vi "SetRampRates_ReadField.vi"(0 "Max Ramp Rate - Z Axis (A/s)":dbl, 1 "Max Ramp Rate - Y Axis (A/s)":dbl, 2 "User defined Ramp Rate (T/min) 2":bool, 3 "User defined Ramp Rate (T/min)":dbl, 5 "Within Limits?":bool, 7 "Y-Axis Field (kG)":dbl, 9 "Z-Axis Field (kG) in":dbl, 11 "error in (no error)":T1, 12 "Y-Axis Communications Config":T2, 13 "Z-Axis Communications Config":T2) -> (4 "All Instruments Responded?":bool, 6 "Current Magnetic\nField\n(430 TCP reading)":T3 {"phi (deg)" format="%#_3g"}, 8 "Ramp Rate along Vector (T/min)":dbl, 10 "Y-Axis Ramp Rate (T/min)":dbl format="%.3f", 14 "Z-Axis Ramp Rate (T/min)":dbl format="%.3f", 15 "error out":T1)   [LabVIEW 2013]
uses:
  VTI LabView IS - Kopie2/devices/magnet/AMI reading polar field.ctl
  VTI LabView IS - Kopie2/app/app global state actions.ctl
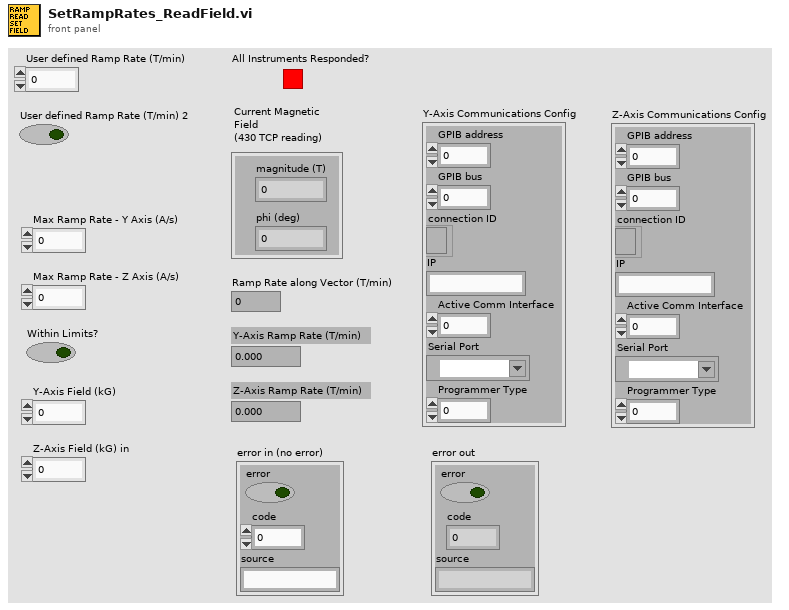
[diagram p1: front panel]
types:
  T1 = cluster{"error":bool, "code":i32, "source":string}
  T2 = cluster{"GPIB address":i16, "GPIB bus":i16, "connection ID":refnum<k5>, "IP":string, "Active Comm Interface":u16, "Serial Port":refnum<visa-resource-name>, "Programmer Type":u16}
  T3 = typedef "AMI reading polar field.ctl" = cluster{"magnitude (T)":dbl, "phi (deg)":dbl}
  T4 = typedef "app global state actions.ctl" = enum16{"set field reached", "get cluster", "set cluster", "set current sweep", "set field value", "set 430 TCP reading", "set ramping", "set sweeping", "append log", "clear log", "set finished"}
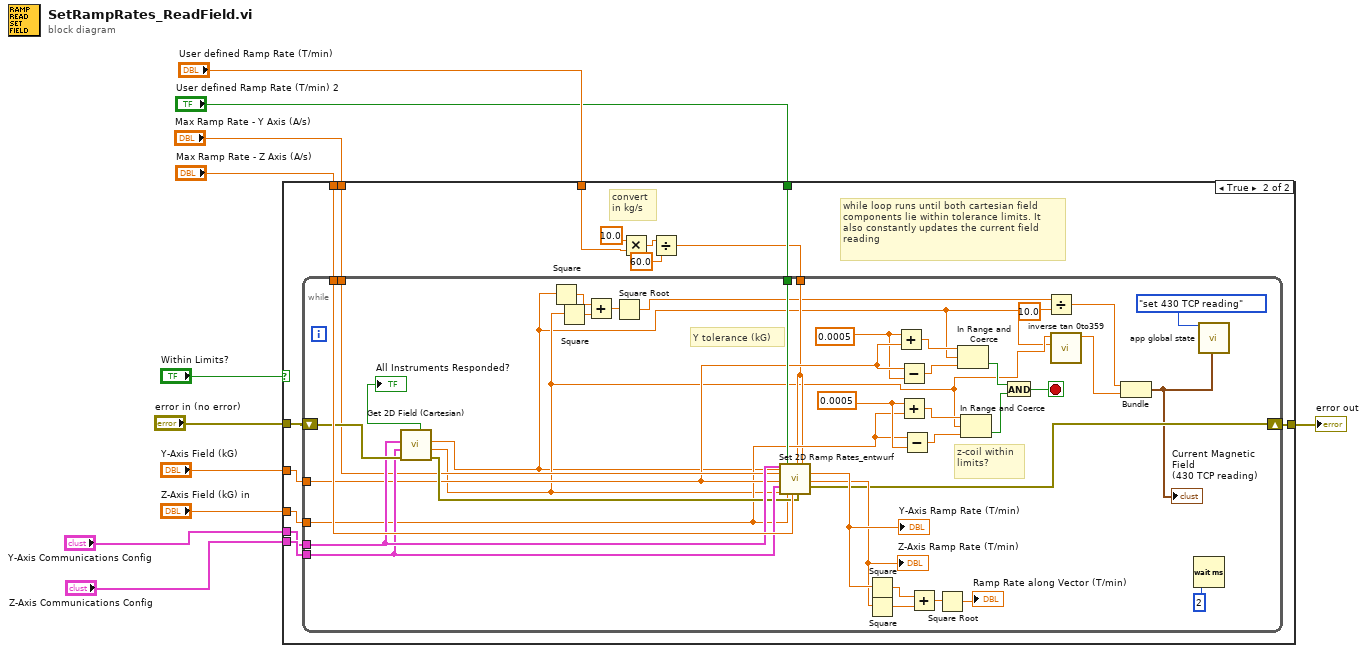
[diagram p0: block diagram]
diagram:
  n1 = case shown="True" "Within Limits?" {
    tunnel: "Z-Axis Field (kG) in" -> [_ w26]
    tunnel: "Y-Axis Field (kG)" -> [_ w25]
    tunnel: [w12 w24] -> w4
    tunnel: "User defined Ramp Rate (T/min) 2" -> [_ w23]
    tunnel: "Max Ramp Rate - Y Axis (A/s)" -> [_ w22]
    tunnel: "Max Ramp Rate - Z Axis (A/s)" -> [_ w21]
    tunnel: "error in (no error)" -> [w12 w20]
    tunnel: "Z-Axis Communications Config" -> [_ w19]
    tunnel: "Y-Axis Communications Config" -> [_ w18]
    tunnel: "User defined Ramp Rate (T/min)" -> [_ w14]
    frame False {
    }
    frame True {
      # "convert \nin kg/s"
      # "while loop runs until both cartesian field components lie within tolerance limits. It also constantly updates the current field reading"
      n2 = Multiply(x=10.0, y=w14) -> (x*y=w16:dbl)
      n3 = Divide(x=w16, y=60.0 ("x")) -> (x/y=w13:dbl)
      n4 = while {
        tunnel: w26 -> [w40]
        tunnel: w25 -> [w44]
        tunnel: w13 -> [w33]
        tunnel: w23 -> [w47]
        shift-right: [w57] -> w24
        shift-left: w20 -> [w56]
        tunnel: w22 -> [w48]
        tunnel: w21 -> [w58]
        tunnel: w19 -> [w54]
        tunnel: w18 -> [w55]
        stop <- w37 stop-if-true
        w34 = 0.0005 ("Y Tolerance (kG)")
        w41 = 0.0005 ("Z Tolerance (kG)")
        # "Y tolerance (kG)"
        # "z-coil within limits?"
        n5 = call <userlib>:"Get 2D Field (Cartesian).vi"("Y-Axis Communications Config"=w55, "Z-Axis Communications Config"=w54, "error in"=w56) -> ("All Instruments Responded?"=→"All Instruments Responded?":bool, "Y-Axis Field (kG)"=w27:dbl, "Z-Axis Field (kG)"=w28:dbl, "error out"=w53:T1)  [unwired: 2 in]
        n6 = Square(x=w27) -> (x^2=w50:dbl)
        n7 = Square(x=w28) -> (x^2=w51:dbl)
        n8 = Add(x=w50, y=w51) -> (x+y=w49:dbl)
        n9 = Square Root(x=w49) -> (sqrt(x)=w29:dbl)
        n10 = call <userlib>:"Set 2D Ramp Rates_entwurf.vi"("Y-Axis Communications Config"=w55, "Y-Axis Field (kG)"=w27, "Next Y-Axis Field (kG)"=w44, "Z-Axis Communications Config"=w54, "Z-Axis Field (kG)"=w28, "User defined Ramp Rate (T/min)"=w47, "Next Z-Axis Field (kG)"=w40, "Max Ramp Rate - Y Axis (A/s)"=w48, "Max Ramp Rate - Z Axis (A/s)"=w58, "User defined Ramp Rate - Z Axis (kG/s)"=w33, "error in"=w53, "User defined Ramp Rate Y-Axis (kG/s)"=w33) -> ("Y-Axis Ramp Rate (T/min)"=w65:dbl, "Z-Axis Ramp Rate (T/min)"=w64:dbl, "error out"=w57:T1)  [unwired: 5 in]
        "Y-Axis Ramp Rate (T/min)" <- w65
        "Z-Axis Ramp Rate (T/min)" <- w64
        n11 = Square(x=w65) -> (x^2=w62:dbl)
        n12 = Square(x=w64) -> (x^2=w63:dbl)
        n13 = Add(x=w34, y=w44) -> (x+y=w46:dbl)
        n14 = Subtract(x=w44, y=w34) -> (x-y=w45:dbl)
        n15 = Add(x=w41, y=w40) -> (x+y=w43:dbl)
        n16 = Subtract(x=w40, y=w41) -> (x-y=w42:dbl)
        n17 = Add(x=w62, y=w63) -> (x+y=w61:dbl)
        n18 = Square Root(x=w61) -> (sqrt(x)=→"Ramp Rate along Vector (T/min)":dbl)
        n19 = In Range and Coerce(upper limit=w46, x=w27, lower limit=w45) -> (In Range?=w39:bool)  [unwired: 1 out]
        n20 = In Range and Coerce(upper limit=w43, x=w28, lower limit=w42) -> (In Range?=w38:bool)  [unwired: 1 out]
        n21 = And(x=w39, y=w38) -> (x .and. y?=w37:bool)
        n22 = Divide(x=w29, y=10.0 ("Y Tolerance (kG)")) -> (x/y=w36:dbl)
        n23 = call "inverse tan 0to359.vi"("y coil"=w27, "z coil"=w28) -> ("phi (deg)"=w30:dbl)  [unwired: 9 in]
        n24 = Bundle(w36, "phi (deg)"=w30) -> (w31:cluster{dbl, "phi (deg)":dbl})  [unwired: 1 in]
        "Current Magnetic\nField\n(430 TCP reading)" <- w31
        n25 = Wait (ms)(milliseconds to wait=2) -> ()  [unwired: 1 out]
        n26 = call "app global state.vi"("action"=app_global_state_actions."set 430 TCP reading" ("app global state actions"), "Current Magnetic Field\n(430 TCP reading)"=w31) -> ()  [unwired: 17 in, 1 out]
      }
    }
  }
  "error out" <- w4
